vi "Purge Water Sequence SM.vi"(0 "Degree Setting":dbl=58.0, 1 "Equipment":T4={"COM Port"="COM9", "MW100"="MW100", "AG34970"="A-34972A", "Chamber"="WT500"}, 2 "Semiphore":T3, 5 "Flow rate setting":dbl=1.5, 7 "Temp Band(+/- F)":dbl=2.0, 9 "Valve Bank":u16(ring) items=["A", "B", "C", "D"], 11 "Error In":errorcluster, 12 "Flow Chart Ref":refnum<vi>, 13 "Temp Chart Ref":refnum<vi>, 14 "Test Condition":T1=enum."Global, Purge") -> (3 "Failed to Start Count":dbl, 4 "Downspout Flow":dbl=2.9, 6 "Downspout Temp":dbl=57.8, 8 "Flow rate setting out":dbl=2.250000000000002, 10 "Temp Setting Out":dbl=61.459999999999994, 15 "Error Out":errorcluster)   [LabVIEW 2012]
uses:
  EquipReferences.ctl
  Cluster Purge Settings.ctl
  TestedFlowratesScenarios.ctl
  ChannelSettings.ctl
  ValveBankPositions.ctl
  Intellifaucet/Intellfaucet Mode.ctl
  HEWH Error Enumeration.ctl
  Global HEWH.vi
panel:
  in  "Stop Chart":bool
  in  "Chart Data":bool
  out "Cold Flow":dbl[](array[numeric])
  in  "Purge Min Time":u32=30
  in  "Failed to Start Limit":dbl=5.0
  out "Output (Percent,GPM)":dbl
  in  "stop":bool
  in  "Ramp Down Array":dbl[](array[numeric])=[2.7, 2.5, 2.3, 2.1, 1.9, 1.7, 1.5, 1.3, 1.1, 0.9, 0.8]
  in  "Purge Settings Cluster":T2={"Temp SettleTimeLimit(S)"=120.0, "Steady State Persist Time(mS)"=30000, "Purge Min Time"=30, "Flow SettleTimeLimit(S)"=120.0, "Flow Adjust Time (3s)"=1.5, "Flow Band (+/-GPM)"=0.25, "Proportional Control Adjust Rate"=0.2}
  out "FlowSetTime":dbl=46.09375
  out "FlowSetStartTime":dbl=60.796875
  out "Settle Time Start":dbl format="%.2f"
  out "FlowErrors":bool[](array[boolean])=[TRUE, TRUE, TRUE, TRUE, TRUE, TRUE, TRUE, TRUE, TRUE, TRUE, TRUE, TRUE, TRUE, TRUE, TRUE, TRUE, TRUE, TRUE, TRUE, TRUE, TRUE, TRUE, TRUE, TRUE, TRUE, TRUE, TRUE, TRUE, TRUE, TRUE, TRUE, TRUE, TRUE, TRUE, TRUE, TRUE, TRUE, TRUE, TRUE, TRUE]
  out "TempErrors":bool[](array[boolean])=[TRUE, TRUE, TRUE, TRUE, TRUE, TRUE, TRUE, TRUE, TRUE, TRUE, TRUE, TRUE, TRUE, TRUE, TRUE, TRUE, TRUE, TRUE, TRUE, TRUE, TRUE, TRUE, TRUE, TRUE, TRUE, TRUE, TRUE, TRUE, TRUE, TRUE, TRUE, TRUE, TRUE, TRUE, TRUE, TRUE, TRUE, TRUE, TRUE, TRUE]
  out "TempSet Time (sec)":dbl=60.015625 format="%.2f"
  in  "Sample Period(mS)":u32=500
  in  "Steady State Persist Time(mS)":u32=20000
  in  "Flow Adjust Time (3s)":dbl=2.0
  in  "Flow SettleTimeLimit(S)":dbl=300.0
  out "Downspout Flow Chart":dbl(graph)=2.9
  out "Current State":string="Finish"
  out "Downspout Temp Chart":dbl(graph)=57.8
  out "-E":dbl=0.10000000000000009
  in  "Proportional Control Adjust Rate":dbl=0.1
  in  "Temp SettleTimeLimit(S)":dbl=300.0
  in  "Flow Band (+/-GPM)":dbl=0.25
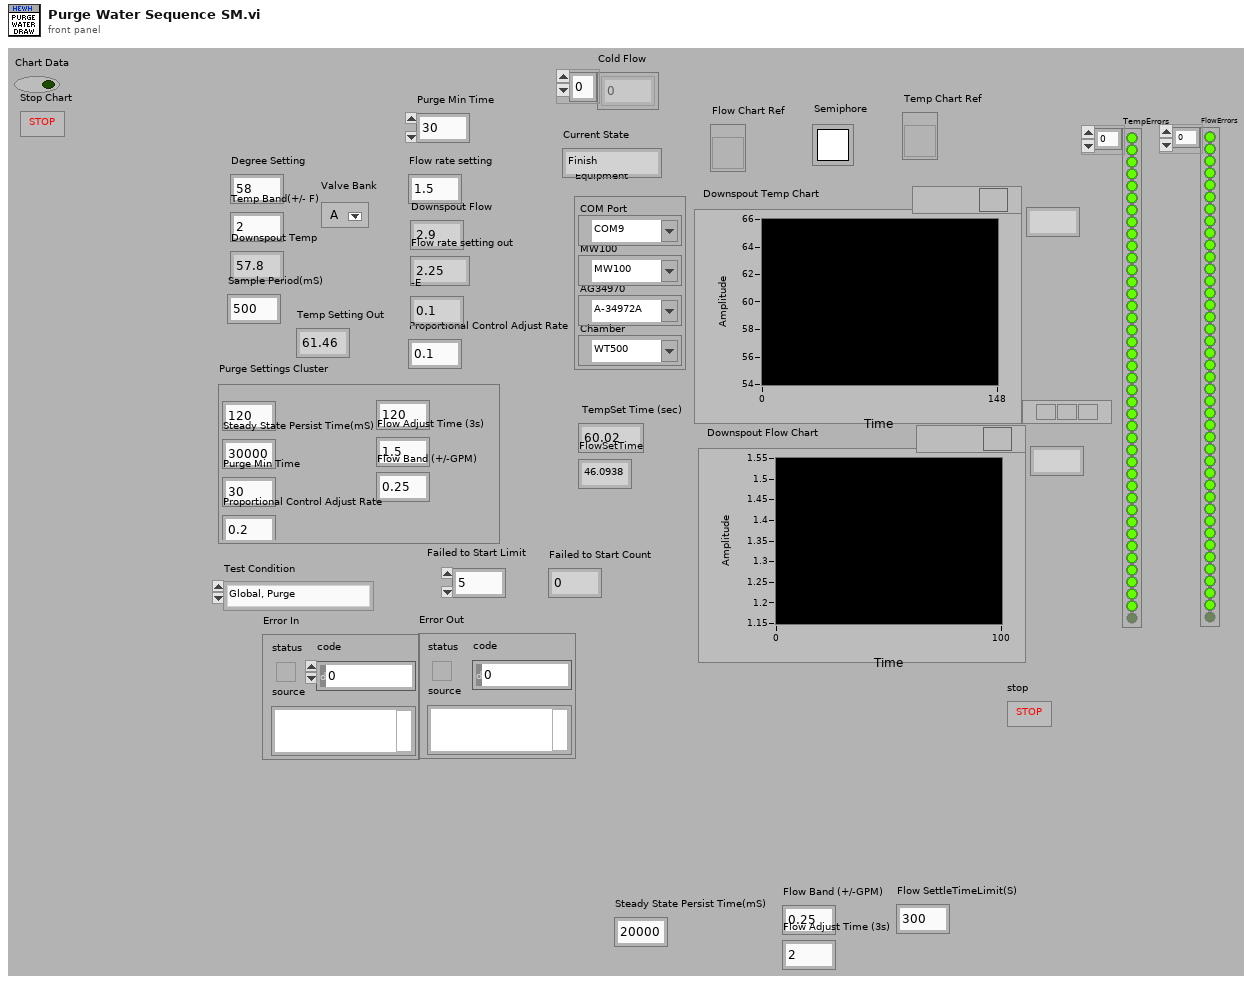
[diagram p1: front panel]
types:
  T1 = typedef "TestedFlowratesScenarios.ctl" = enum16{"DRK500,Station1", "DRK375,Lab", "SRK500,Station1,5GPM FR", "DRK375,STATION3,1/2\"HOSE", "DRK500,Station1,downspout", "DRK375,Station3,thruEcocute", "DRK375,Station3,purge", "Build2,2B,Purge", "Global, Purge", "Global, Tank"}
  T2 = typedef "Cluster Purge Settings.ctl" = cluster{"Temp SettleTimeLimit(S)":dbl, "Steady State Persist Time(mS)":u32, "Purge Min Time":i32, "Flow SettleTimeLimit(S)":dbl, "Flow Adjust Time (3s)":dbl, "Flow Band (+/-GPM)":dbl, "Proportional Control Adjust Rate":dbl}
  T3 = typedef "Semaphore RefNum" = refnum<k1>
  T4 = typedef "EquipReferences.ctl" = cluster{"COM Port":refnum<visa-resource-name>, "MW100":refnum<visa-resource-name>, "AG34970":refnum<visa-resource-name>, "Chamber":refnum<visa-resource-name>}
  T5 = typedef "ValveBankPositions.ctl" = enum16{"Heating", "Purge", "Resting", "Draw"}
  T6 = typedef "HEWH Error Enumeration.ctl" = enum16{"No Error", "GEA2 Send ACK Mismatch", "GEA2 STX", "GEA2 ETX", "GEA2 CRC Mismatch", "GEA2 ReadACK", "RTD In Range Error", "Fail Mean Tank Temp", "No Flow Config Data Found", "Failed Flow During Purge", "Temp During Purge", "Confirm IF Stop Fail", "Init Draw: TC_1 Out of Range", "Flow = 0 During Draw after 20s"}
  T7 = typedef "Intellfaucet Mode.ctl" = enum16{"Adjust Temp", "Adjust Flow", "Start Flow", "Stop Flow"}
  T8 = typedef "ChannelSettings.ctl" = u32
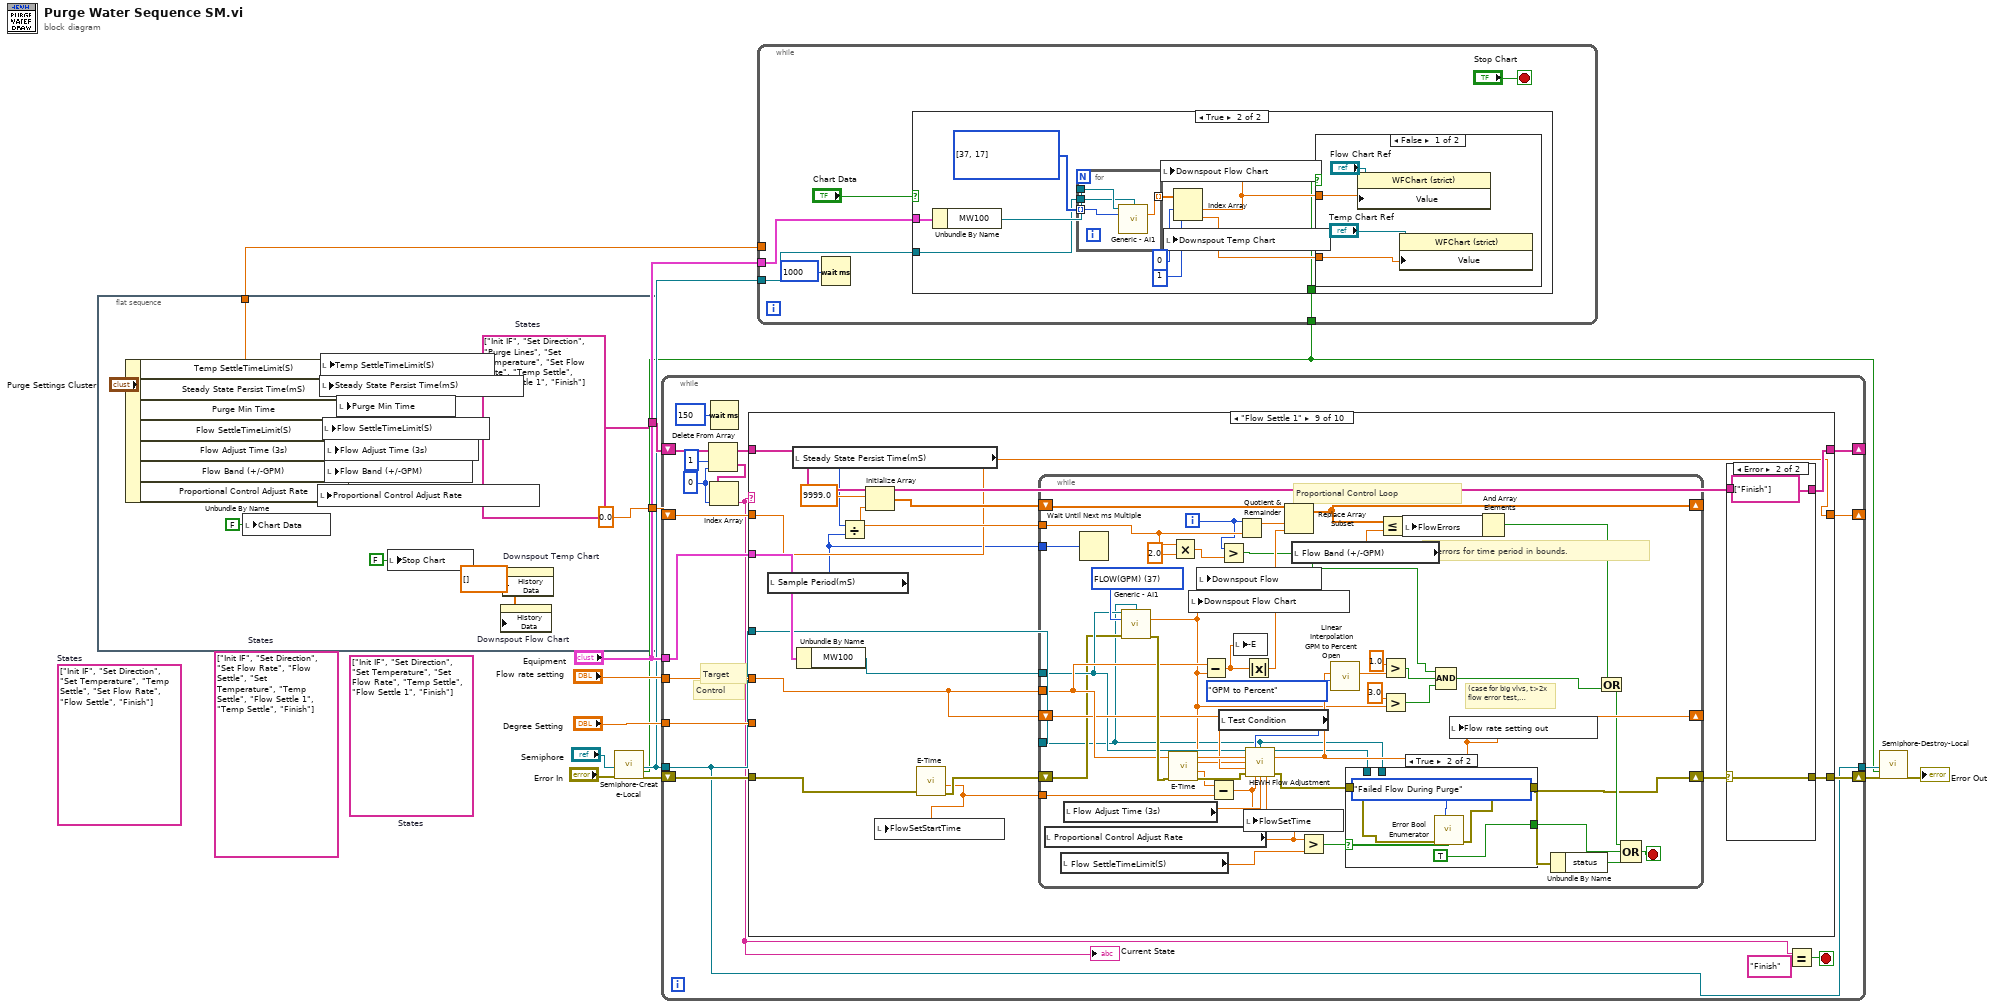
[diagram p0: block diagram]
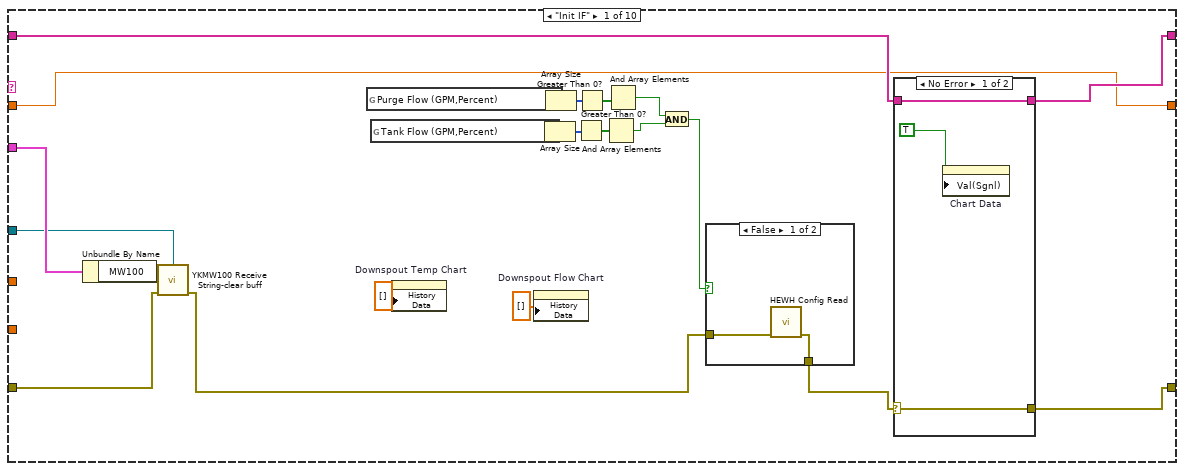
[diagram p4: hidden frame]
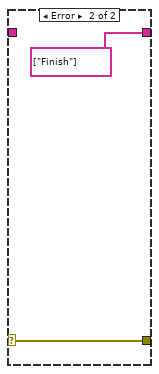
[diagram p6: hidden frame]
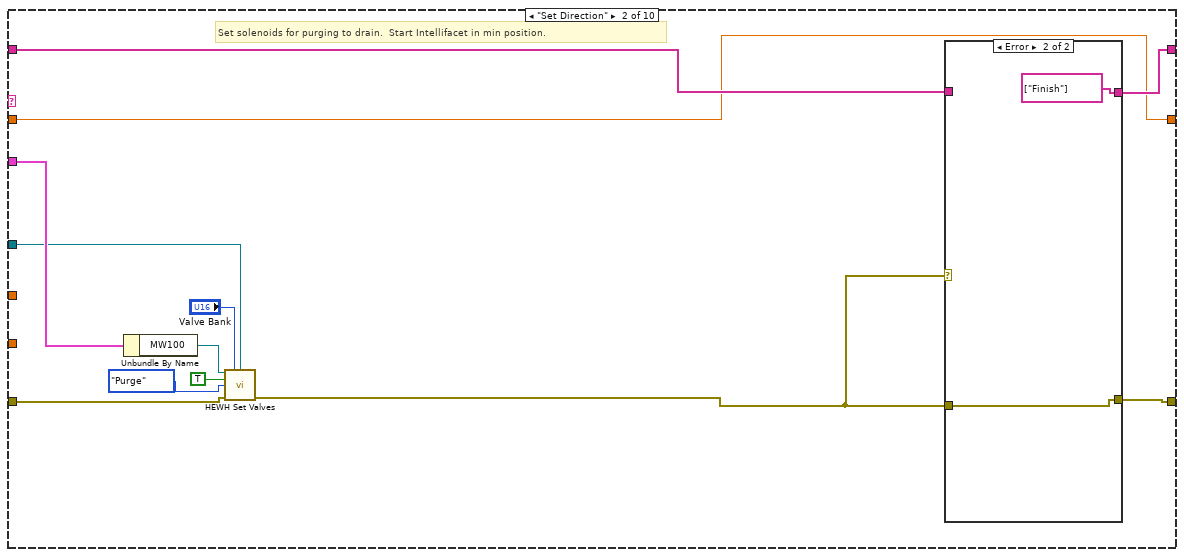
[diagram p7: hidden frame]
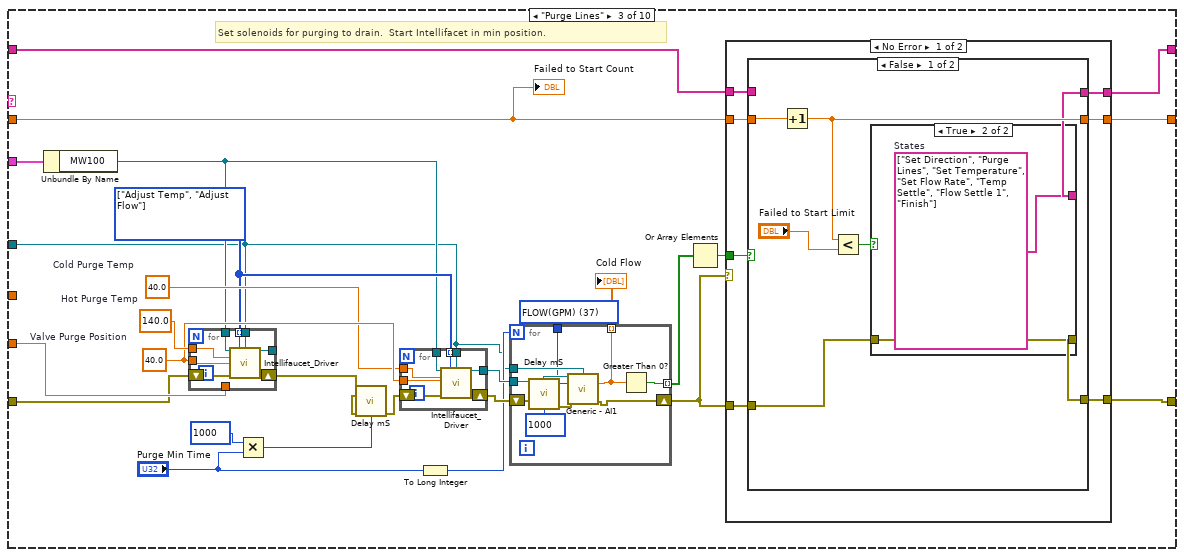
[diagram p9: hidden frame]
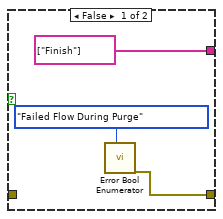
[diagram p10: hidden frame]
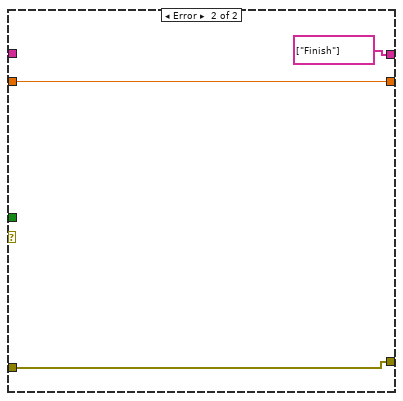
[diagram p12: hidden frame]
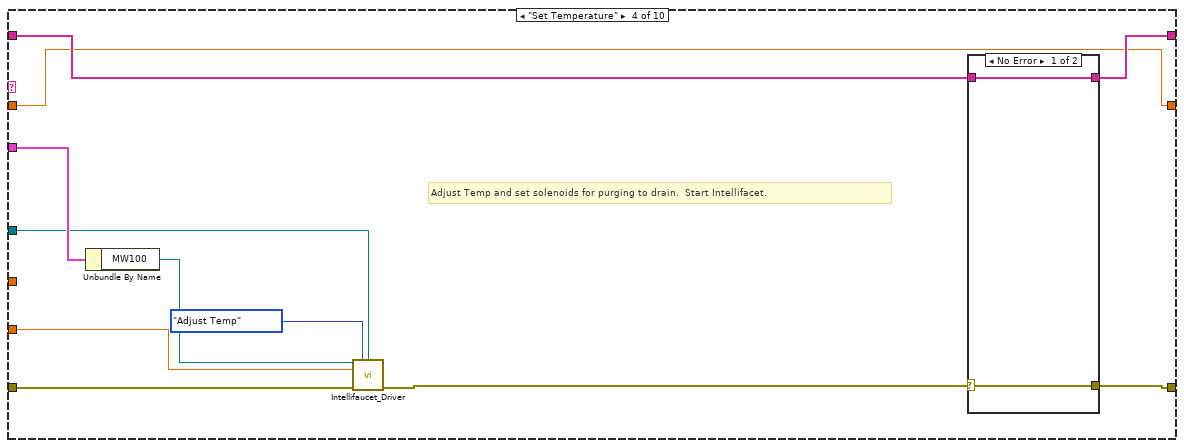
[diagram p13: hidden frame]
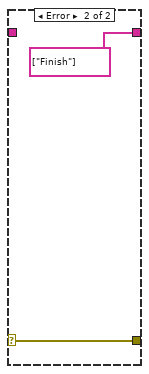
[diagram p14: hidden frame]
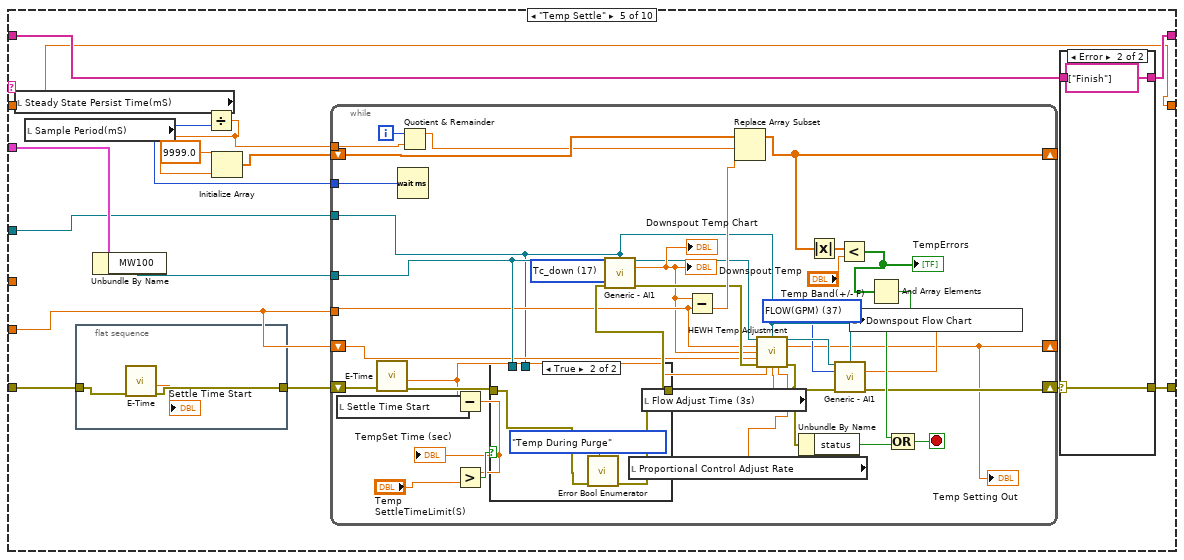
[diagram p15: hidden frame]
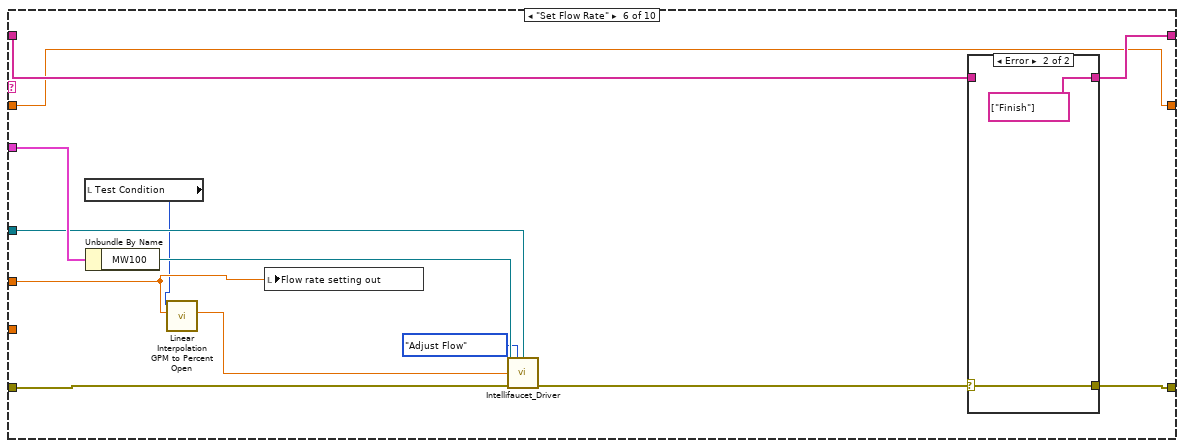
[diagram p18: hidden frame]
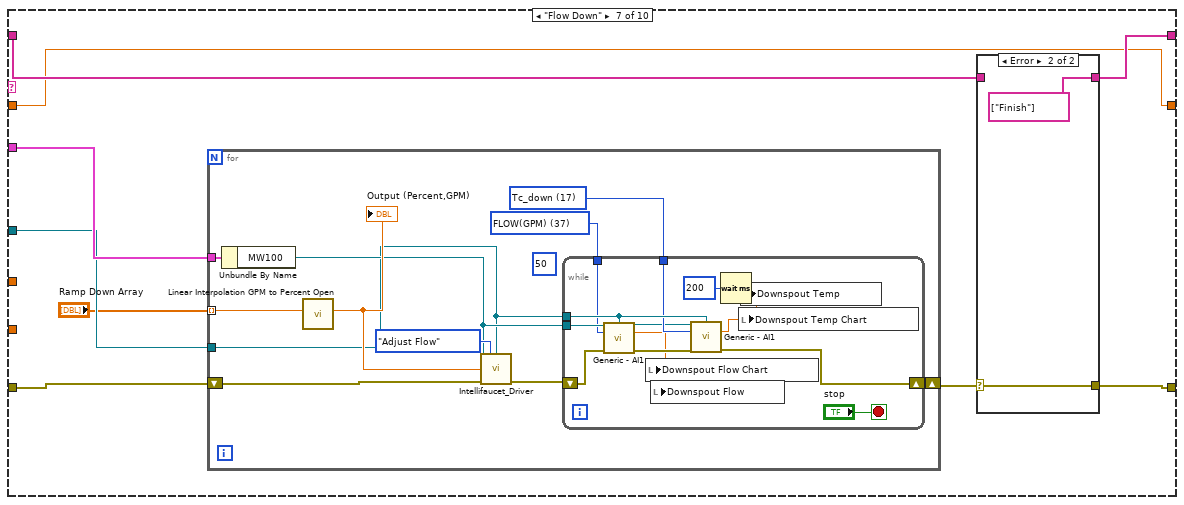
[diagram p20: hidden frame]
diagram:
  (unwired) string[] ["Init IF", "Set Direction", "Set Temperature", "Set Flow Rate", "Temp Settle", "Flow Settle 1", "Finish"]  # States
  (unwired) string[] ["Init IF", "Set Direction", "Set Flow Rate", "Flow Settle", "Set Temperature", "Temp Settle", "Flow Settle 1", "Temp Settle", "Finish"]  # States
  (unwired) string[] ["Init IF", "Set Direction", "Set Temperature", "Temp Settle", "Set Flow Rate", "Flow Settle", "Finish"]  # States
  n1 = flat-sequence {
    tunnel: [w19] -> w14
    tunnel: [0.0] -> w5
    tunnel: [w15] -> w1
    frame #0 {
      w19 = string[] ["Init IF", "Set Direction", "Purge Lines", "Set Temperature", "Set Flow Rate", "Temp Settle", "Flow Settle 1", "Finish"]  # States
      w20 = dbl[] [] ("History Data")
      n2 = Unbundle By Name("Purge Settings Cluster") -> ("Temp SettleTimeLimit(S)"=w15:dbl, "Steady State Persist Time(mS)"=w27:u32, "Purge Min Time"=w18:i32, "Flow SettleTimeLimit(S)"=w26:dbl, "Flow Adjust Time (3s)"=w25:dbl, "Flow Band (+/-GPM)"=w24:dbl, "Proportional Control Adjust Rate"=w23:dbl)
      n3 = local write "Chart Data"(FALSE ("Chart Data")) -> ()
      n4 = local write "Proportional Control Adjust Rate"(w23) -> ()
      n5 = local write "Steady State Persist Time(mS)"(w27) -> ()
      n6 = local write "Temp SettleTimeLimit(S)"(w15) -> ()
      n7 = local write "Flow SettleTimeLimit(S)"(w26) -> ()
      n8 = local write "Flow Adjust Time (3s)"(w25) -> ()
      n9 = local write "Flow Band (+/-GPM)"(w24) -> ()
      n10 = local write "Purge Min Time"(w18) -> ()
      n11 = local write "Stop Chart"(FALSE ("Stop Chart")) -> ()
      n12 = property on="Downspout Flow Chart" class="WFChart (strict)"("History Data"=w20) -> ()  [unwired: 2 in, 2 out]
      n13 = property on="Downspout Temp Chart" class="WFChart (strict)"("History Data"=w20) -> ()  [unwired: 2 in, 2 out]
    }
  }
  n14 = call "Semiphore-Create-Local.vi"("Semiphore"="Semiphore", "error in (no error)"="Error In") -> ("semaphore"=w3:T3, "Local?"=w2:bool, "error out"=w10:errorcluster)  [unwired: 15 in]
  n15 = while {
    shift-right: [w41] -> _
    shift-left: w14 -> [w45]
    shift-right: [w38] -> w9
    shift-left: w10 -> [w37]
    tunnel: "Equipment" -> [w30]
    tunnel: "Degree Setting" -> [w34]
    tunnel: "Flow rate setting" -> [w33]
    tunnel: w3 -> [w29]
    tunnel: [w29] -> w7
    shift-right: [w32] -> _
    shift-left: w5 -> [w31]
    stop <- w36 stop-if-true
    w42 = 0 ("index")
    # "Control"
    # "Target"
    n16 = Delete From Array(array=w45, length=1, index=w42) -> (deleted portion=w43:string[], array with subset deleted=w40:string[])
    n17 = Index Array(array=w43, index=w42) -> (element=w28:string)
    "Current State" <- w28
    n18 = Wait (ms)(milliseconds to wait=u32 150) -> ()  [unwired: 1 out]
    n19 = case shown="\"Flow Settle 1\"" w28 {
      tunnel: [w61 w85 w116 w176 w195 w257 w270 w315 w386 w451] -> w41
      tunnel: w40 -> [w62 w86 w117 w177 w196 w258 w271 w316 w387 w450]
      tunnel: [w59 w84 w115 w175 w193 w256 w269 w313 w384 w449] -> w38
      tunnel: w37 -> [w64 w83 w109 w174 w190 w254 w267 w311 w382 w448]
      tunnel: w30 -> [w66 w82 w92 w178 w198 w259 w272 w317 w388 _]
      tunnel: w34 -> [_ _ w110 w173 w184 _ _ _ _ _]
      tunnel: w33 -> [_ _ _ _ _ w248 _ w310 w372 _]
      tunnel: w29 -> [w63 w79 w91 w169 w192 w252 w266 w303 w377 _]
      tunnel: [w60 w76 w113 w168 w183 w249 w265 w301 w375 w447] -> w32
      tunnel: w31 -> [w60 w76 w111 w168 w183 w249 w265 w301 w375 w447]
      frame "Init IF" {
        n20 = Unbundle By Name(w66) -> ("MW100"=w65:refnum<visa-resource-name>)
        n21 = call "YKMW100 Receive String-clear buff.vi"("VISA session"=w65, "Semiphore"=w63, "error in (no error)"=w64) -> ("error out"=w48:errorcluster)  [unwired: 10 in, 2 out]
        n22 = global read "Global HEWH.vi" "Purge Flow (GPM,Percent)"() -> (w58:dbl[][])
        n23 = global read "Global HEWH.vi" "Tank Flow (GPM,Percent)"() -> (w57:dbl[][])
        n24 = property on="Downspout Temp Chart" class="WFChart (strict)"("History Data"=dbl[] []) -> ()  [unwired: 2 in, 2 out]
        n25 = property on="Downspout Flow Chart" class="WFChart (strict)"("History Data"=dbl[] []) -> ()  [unwired: 2 in, 2 out]
        n26 = Array Size(array=w57) -> (size(s)=w55:i32[])
        n27 = Array Size(array=w58) -> (size(s)=w56:i32[])
        n28 = Greater Than 0?(x=w55) -> (x > 0?=w53:bool[])
        n29 = Greater Than 0?(x=w56) -> (x > 0?=w54:bool[])
        n30 = And Array Elements(Boolean array=w53) -> (logical AND=w51:bool)
        n31 = And Array Elements(Boolean array=w54) -> (logical AND=w52:bool)
        n32 = And(x=w52, y=w51) -> (x .and. y?=w50:bool)
        n33 = case shown="False" w50 {
          tunnel: w48 -> [w68 w69]
          tunnel: [w67 w69] -> w49
          frame False {
            n34 = call "HEWH Config Read.vi"("error in (no error)"=w68) -> ("error out"=w67:errorcluster)  [unwired: 13 in, 1 out]
          }
          frame True {
          }
        }
        n35 = case shown="No Error" w49 {
          selector: w49 -> [w71 w74]
          tunnel: [w72 string[] ["Finish"] ("States")] -> w61
          tunnel: w62 -> [w72 _]
          tunnel: [w71 w74] -> w59
          frame No Error {
            n36 = property on="Chart Data" class="Bool (strict)"("Val(Sgnl)"=TRUE ("Chart Data")) -> ()  [unwired: 2 in, 2 out]
          }
          frame Error {
          }
        }
      }
      frame "Set Direction" {
        # "Set solenoids for purging to drain.  Start Intellifacet in min position."
        n37 = Unbundle By Name(w82) -> ("MW100"=w81:refnum<visa-resource-name>)
        n38 = call "HEWH Set Valves.vi"("VISA session"=w81, "Valve Bank"="Valve Bank", "Semiphore"=w79, "Expansion Tank?"=TRUE, "Valve Bank Setting"=ValveBankPositions."Purge", "Error In"=w83) -> ("Error Out"=w75:errorcluster)  [unwired: 8 in, 1 out]
        n39 = case shown="Error" w75 {
          tunnel: w86 -> [w88 _]
          tunnel: [w88 string[] ["Finish"] ("States")] -> w85
          tunnel: [w87 w89] -> w84
          tunnel: w75 -> [w87 w89]
          frame No Error {
          }
          frame Error {
          }
        }
      }
      frame "Purge Lines" {
        w99 = 40.0  # Cold Purge Temp
        w100 = 40.0  # Valve Purge Position
        w108 = 140.0  # Hot Purge Temp
        w98 = T7[] [enum."Adjust Temp", enum."Adjust Flow"] items=["Adjust Temp", "Adjust Flow", "Start Flow", "Stop Flow"]
        w114 = T8 37 items=["4-20_OUT", "Pres_HI1", "Pres_HI2", "Pres_LOW", "Pres_PIN", "HEATER_TOP", "HEATER_BOT", "T_Shell", "FLOWMETER", "WATT_SENSE", "WH_TICK", "Tc_1", "Tc_2", "Tc_3", "Tc_4", "Tc_5", "Tc_6", "Tc_down", "T_Shell_2", "T_Shell_3", "T_Shell_4", "RTD_IN", "RTD_OUT", "RTD_AMB", "INTF_TEMPFLO", "INTF_READY", "INTF_START", "INTF_STOP", "DRM_LOW", "DRM_HIGH", "PWR_MAIN", "VLV_DUMP", "VLV_OUT", "VLV_IN", "WATT_HOURS", "FLOW(SAMPLE)", "GALLONS", "FLOW(GPM)"] ("Channel_Enum")
        # "Set solenoids for purging to drain.  Start Intellifacet in min position."
        n40 = Unbundle By Name(w92) -> ("MW100"=w93:refnum<visa-resource-name>)
        n41 = for {
          tunnel: [w133] -> _
          tunnel: w98 -> [w132] mode=indexing
          tunnel: w91 -> [w129]
          shift-right: [w131] -> w107
          shift-left: w109 -> [w130]
          tunnel: w93 -> [w128]
          tunnel: w110 -> [_]
          tunnel: w100 -> [w126]
          tunnel: w108 -> [w127]
          n42 = call "Intellifaucet_Driver.vi"("VISA session"=w128, "Mode"=w132, "Semiphore"=w129, "Temperature(F)"=w127, "Percent Flow"=w126, "Error In"=w130) -> ("VISA session out"=w133:refnum<visa-resource-name>, "Error Out"=w131:errorcluster)  [unwired: 8 in]
        }
        n43 = Multiply(x=u32 1000 ("milliseconds to wait"), y="Purge Min Time") -> (x*y=w104:u32)
        n44 = call "Delay mS.vi"("Error In"=w107, "milliseconds to wait"=w104) -> ("Error Out"=w103:errorcluster)  [unwired: 13 in]
        n45 = for {
          tunnel: [w125] -> w101
          tunnel: w98 -> [w124] mode=indexing
          tunnel: w91 -> [w121]
          shift-right: [w123] -> w102
          shift-left: w103 -> [w122]
          tunnel: w93 -> [w120]
          tunnel: w100 -> [w119]
          tunnel: w99 -> [w118]
          n46 = call "Intellifaucet_Driver.vi"("VISA session"=w120, "Mode"=w124, "Semiphore"=w121, "Temperature(F)"=w118, "Percent Flow"=w119, "Error In"=w122) -> ("VISA session out"=w125:refnum<visa-resource-name>, "Error Out"=w123:errorcluster)  [unwired: 8 in]
        }
        n47 = To Long Integer(number="Purge Min Time") -> (32bit integer=w97:i32)
        n48 = for {
          N: w97 -> [_]
          tunnel: w91 -> [w140]
          tunnel: w101 -> [w139]
          tunnel: w114 -> [w138]
          tunnel: [w137] -> w96 mode=indexing
          shift-right: [w136] -> w112
          shift-left: w102 -> [w142]
          tunnel: [w134] -> w94 mode=indexing
          n49 = call "Delay mS.vi"("Error In"=w142, "milliseconds to wait"=u32 1000) -> ("Error Out"=w141:errorcluster)  [unwired: 13 in]
          n50 = call "Generic - AI1.vi"("MW100"=w139, "Semiphore"=w140, "Channel_Enum"=w138, "Error In"=w141) -> ("Value"=w134:dbl, "Error Out"=w136:errorcluster)  [unwired: 9 in, 1 out]
          n51 = Greater Than 0?(x=w134) -> (x > 0?=w137:bool)
        }
        "Cold Flow" <- w94
        n52 = Or Array Elements(Boolean array=w96) -> (logical OR=w95:bool)
        n53 = case shown="No Error" w112 {
          tunnel: w117 -> [w149 _]
          tunnel: [w148 string[] ["Finish"] ("States")] -> w116
          tunnel: [w147 w165] -> w115
          tunnel: w112 -> [w146 w165]
          tunnel: w95 -> [w145 _]
          tunnel: [w144 w166] -> w113
          tunnel: w111 -> [w143 w166]
          frame No Error {
            n54 = case shown="False" w145 {
              tunnel: w149 -> [_ w164]
              tunnel: [w152 w164] -> w148
              tunnel: [w151 w162] -> w147
              tunnel: w146 -> [w150 w162]
              tunnel: [w155 w163] -> w144
              tunnel: w143 -> [w156 w163]
              frame False {
                n55 = Increment(x=w156) -> (x+1=w155:dbl)
                n56 = Less?(x=w155, y="Failed to Start Limit") -> (x < y?=w153:bool)
                n57 = case shown="True" w153 {
                  tunnel: [string[] ["Finish"] ("States") w160] -> w152
                  tunnel: [w158 w161] -> w151
                  tunnel: w150 -> [_ w161]
                  frame False {
                    n58 = call "Error Bool Enumerator.vi"("Error Enum"=HEWH_Error_Enumeration."Failed Flow During Purge") -> ("Error Out"=w158:errorcluster)  [unwired: 8 in]
                  }
                  frame True {
                    w160 = string[] ["Set Direction", "Purge Lines", "Set Temperature", "Set Flow Rate", "Temp Settle", "Flow Settle 1", "Finish"]  # States
                  }
                }
              }
              frame True {
              }
            }
          }
          frame Error {
          }
        }
        "Failed to Start Count" <- w111
      }
      frame "Set Temperature" {
        # "Adjust Temp and set solenoids for purging to drain.  Start Intellifacet."
        n59 = Unbundle By Name(w178) -> ("MW100"=w171:refnum<visa-resource-name>)
        n60 = call "Intellifaucet_Driver.vi"("VISA session"=w171, "Mode"=Intellfaucet_Mode."Adjust Temp", "Semiphore"=w169, "Temperature(F)"=w173, "Error In"=w174) -> ("Error Out"=w170:errorcluster)  [unwired: 9 in, 1 out]
        n61 = case shown="No Error" w170 {
          selector: w170 -> [w179 w182]
          tunnel: [w180 string[] ["Finish"] ("States")] -> w176
          tunnel: w177 -> [w180 _]
          tunnel: [w179 w182] -> w175
          frame No Error {
          }
          frame Error {
          }
        }
      }
      frame "Temp Settle" {
        n62 = local read "Steady State Persist Time(mS)"() -> (w189:u32)
        n63 = local read "Sample Period(mS)"() -> (w185:u32)
        n64 = flat-sequence {
          tunnel: [w201] -> w191
          tunnel: w190 -> [w200]
          frame #0 {
            n65 = call "E-Time.vi"("error in (no error)"=w200) -> ("error out"=w201:errorcluster, "Elapsed Time (sec)"=→"Settle Time Start":dbl)  [unwired: 8 in, 1 out]
          }
        }
        n66 = Unbundle By Name(w198) -> ("MW100"=w197:refnum<visa-resource-name>)
        n67 = Divide(x=w189, y=w185) -> (x/y=w187:dbl)
        n68 = Initialize Array(9999.0 ("element"), w187) -> (w186:dbl[])
        n69 = while {
          tunnel: w197 -> [w221]
          tunnel: w184 -> [w219]
          shift-right: [w212] -> w194
          shift-left: w191 -> [w227]
          tunnel: w192 -> [w210]
          tunnel: w187 -> [w237]
          shift-right: [w233] -> _
          shift-left: w186 -> [w236]
          tunnel: w185 -> [w228]
          shift-right: [w206] -> _
          shift-left: w184 -> [w217]
          i -> [w238]
          stop <- w242 stop-if-true
          w208 = T8 37 items=["4-20_OUT", "Pres_HI1", "Pres_HI2", "Pres_LOW", "Pres_PIN", "HEATER_TOP", "HEATER_BOT", "T_Shell", "FLOWMETER", "WATT_SENSE", "WH_TICK", "Tc_1", "Tc_2", "Tc_3", "Tc_4", "Tc_5", "Tc_6", "Tc_down", "T_Shell_2", "T_Shell_3", "T_Shell_4", "RTD_IN", "RTD_OUT", "RTD_AMB", "INTF_TEMPFLO", "INTF_READY", "INTF_START", "INTF_STOP", "DRM_LOW", "DRM_HIGH", "PWR_MAIN", "VLV_DUMP", "VLV_OUT", "VLV_IN", "WATT_HOURS", "FLOW(SAMPLE)", "GALLONS", "FLOW(GPM)"] ("Channel_Enum")
          w240 = T8 17 items=["4-20_OUT", "Pres_HI1", "Pres_HI2", "Pres_LOW", "Pres_PIN", "HEATER_TOP", "HEATER_BOT", "T_Shell", "FLOWMETER", "WATT_SENSE", "WH_TICK", "Tc_1", "Tc_2", "Tc_3", "Tc_4", "Tc_5", "Tc_6", "Tc_down", "T_Shell_2", "T_Shell_3", "T_Shell_4", "RTD_IN", "RTD_OUT", "RTD_AMB", "INTF_TEMPFLO", "INTF_READY", "INTF_START", "INTF_STOP", "DRM_LOW", "DRM_HIGH", "PWR_MAIN", "VLV_DUMP", "VLV_OUT", "VLV_IN", "WATT_HOURS", "FLOW(SAMPLE)", "GALLONS", "FLOW(GPM)"] ("Channel_Enum")
          n70 = local read "Settle Time Start"() -> (w223:dbl)
          n71 = call "E-Time.vi"("error in (no error)"=w227) -> ("error out"=w226:errorcluster, "Elapsed Time (sec)"=w216:dbl)  [unwired: 8 in, 1 out]
          n72 = Wait (ms)(milliseconds to wait=w228) -> ()  [unwired: 1 out]
          n73 = Quotient & Remainder(x=w238, y=w237) -> (x-y*floor(x/y)=w235:dbl)  [unwired: 1 out]
          n74 = Subtract(x=w216, y=w223) -> (x-y=w222:dbl)
          "TempSet Time (sec)" <- w222
          n75 = Greater?(x=w222, y="Temp SettleTimeLimit(S)") -> (0:w241:bool)
          n76 = case shown="True" w241 {
            tunnel: w226 -> [w243 w244]
            tunnel: [w243 w245] -> w225
            tunnel: w210 -> [_ _]
            tunnel: w221 -> [_ _]
            frame False {
            }
            frame True {
              n77 = call "Error Bool Enumerator.vi"("Error Enum"=HEWH_Error_Enumeration."Temp During Purge", "Error In"=w244) -> ("Error Out"=w245:errorcluster)  [unwired: 7 in]
            }
          }
          n78 = call "Generic - AI1.vi"("MW100"=w221, "Semiphore"=w210, "Channel_Enum"=w240, "Error In"=w225) -> ("dup VISA session"=w215:refnum<visa-resource-name>, "Value"=w218:dbl, "Error Out"=w220:errorcluster)  [unwired: 9 in]
          "Downspout Temp" <- w218
          "Downspout Temp Chart" <- w218
          n79 = local read "Proportional Control Adjust Rate"() -> (w213:dbl)
          n80 = local read "Flow Adjust Time (3s)"() -> (w214:dbl)
          n81 = Subtract(x=w218, y=w219) -> (x-y=w234:dbl)
          n82 = Replace Array Subset(array=w236, new element=w234, index=w235) -> (w233:dbl[])
          n83 = call "HEWH Temp Adjustment.vi"("VISA session"=w215, "Semiphore"=w210, "Degrees Target(58)"=w219, "Degrees reading"=w218, "Degrees setting In"=w217, "Error In"=w220, "Elapsed Time (sec)"=w216, "Temp Adjust Time (3s)"=w214, "K(0.1)"=w213) -> ("VISA session out"=w209:refnum<visa-resource-name>, "Degree setting Out"=w206:dbl, "Error Out"=w211:errorcluster)  [unwired: 4 in]
          "Temp Setting Out" <- w206
          n84 = Unbundle By Name(w211) -> ("status"=w224:bool)
          n85 = Absolute Value(x=w233) -> (abs(x)=w232:dbl[])
          n86 = call "Generic - AI1.vi"("MW100"=w209, "Semiphore"=w210, "Channel_Enum"=w208, "Error In"=w211) -> ("Value"=w207:dbl, "Error Out"=w212:errorcluster)  [unwired: 9 in, 1 out]
          n87 = Less?(x=w232, y="Temp Band(+/- F)") -> (x < y?=w230:bool[])
          "TempErrors" <- w230
          n88 = local write "Downspout Flow Chart"(w207) -> ()
          n89 = And Array Elements(Boolean array=w230) -> (logical AND=w229:bool)
          n90 = Compound Arithmetic op=OR(w229, w224) -> (w242:bool)
        }
        n91 = case shown="Error" w194 {
          selector: w194 -> [w202 w205]
          tunnel: [w203 string[] ["Finish"] ("States")] -> w195
          tunnel: w196 -> [w203 _]
          tunnel: [w202 w205] -> w193
          frame No Error {
          }
          frame Error {
          }
        }
      }
      frame "Set Flow Rate" {
        n92 = local read "Test Condition"() -> (w247:T1)
        n93 = Unbundle By Name(w259) -> ("MW100"=w253:refnum<visa-resource-name>)
        n94 = call "Linear Interpolation GPM to Percent Open.vi"("Input (GPM,Percent)"=w248, "Configuration"=w247) -> ("Output (Percent,GPM)"=w250:dbl)  [unwired: 9 in]
        n95 = local write "Flow rate setting out"(w248) -> ()
        n96 = call "Intellifaucet_Driver.vi"("VISA session"=w253, "Mode"=Intellfaucet_Mode."Adjust Flow", "Semiphore"=w252, "Percent Flow"=w250, "Error In"=w254) -> ("Error Out"=w255:errorcluster)  [unwired: 9 in, 1 out]
        n97 = case shown="Error" w255 {
          selector: w255 -> [w260 w263]
          tunnel: [w261 string[] ["Finish"] ("States")] -> w257
          tunnel: w258 -> [w261 _]
          tunnel: [w260 w263] -> w256
          frame No Error {
          }
          frame Error {
          }
        }
      }
      frame "Flow Down" {
        n98 = for {
          tunnel: w272 -> [w283]
          tunnel: w266 -> [w277]
          shift-right: [w273] -> w268
          shift-left: w267 -> [w282]
          tunnel: "Ramp Down Array" -> [w279] mode=indexing
          w275 = T8 17 items=["4-20_OUT", "Pres_HI1", "Pres_HI2", "Pres_LOW", "Pres_PIN", "HEATER_TOP", "HEATER_BOT", "T_Shell", "FLOWMETER", "WATT_SENSE", "WH_TICK", "Tc_1", "Tc_2", "Tc_3", "Tc_4", "Tc_5", "Tc_6", "Tc_down", "T_Shell_2", "T_Shell_3", "T_Shell_4", "RTD_IN", "RTD_OUT", "RTD_AMB", "INTF_TEMPFLO", "INTF_READY", "INTF_START", "INTF_STOP", "DRM_LOW", "DRM_HIGH", "PWR_MAIN", "VLV_DUMP", "VLV_OUT", "VLV_IN", "WATT_HOURS", "FLOW(SAMPLE)", "GALLONS", "FLOW(GPM)"] ("Channel_Enum")
          w276 = T8 37 items=["4-20_OUT", "Pres_HI1", "Pres_HI2", "Pres_LOW", "Pres_PIN", "HEATER_TOP", "HEATER_BOT", "T_Shell", "FLOWMETER", "WATT_SENSE", "WH_TICK", "Tc_1", "Tc_2", "Tc_3", "Tc_4", "Tc_5", "Tc_6", "Tc_down", "T_Shell_2", "T_Shell_3", "T_Shell_4", "RTD_IN", "RTD_OUT", "RTD_AMB", "INTF_TEMPFLO", "INTF_READY", "INTF_START", "INTF_STOP", "DRM_LOW", "DRM_HIGH", "PWR_MAIN", "VLV_DUMP", "VLV_OUT", "VLV_IN", "WATT_HOURS", "FLOW(SAMPLE)", "GALLONS", "FLOW(GPM)"] ("Channel_Enum")
          (unwired) 50
          n99 = Unbundle By Name(w283) -> ("MW100"=w278:refnum<visa-resource-name>)
          n100 = call "Linear Interpolation GPM to Percent Open.vi"("Input (GPM,Percent)"=w279) -> ("Output (Percent,GPM)"=w280:dbl)  [unwired: 10 in]
          "Output (Percent,GPM)" <- w280
          n101 = call "Intellifaucet_Driver.vi"("VISA session"=w278, "Mode"=Intellfaucet_Mode."Adjust Flow", "Semiphore"=w277, "Percent Flow"=w280, "Error In"=w282) -> ("Error Out"=w274:errorcluster)  [unwired: 9 in, 1 out]
          n102 = while {
            tunnel: w278 -> [w295]
            tunnel: w277 -> [w294]
            tunnel: w276 -> [w292]
            tunnel: w275 -> [w291]
            shift-right: [w287] -> w273
            shift-left: w274 -> [w289]
            stop <- "stop" stop-if-true
            n103 = call "Generic - AI1.vi"("MW100"=w295, "Semiphore"=w294, "Channel_Enum"=w292, "Error In"=w289) -> ("dup VISA session"=w290:refnum<visa-resource-name>, "Value"=w286:dbl, "Error Out"=w288:errorcluster)  [unwired: 9 in]
            n104 = local write "Downspout Flow Chart"(w286) -> ()
            n105 = local write "Downspout Flow"(w286) -> ()
            n106 = call "Generic - AI1.vi"("MW100"=w290, "Semiphore"=w294, "Channel_Enum"=w291, "Error In"=w288) -> ("Value"=w285:dbl, "Error Out"=w287:errorcluster)  [unwired: 9 in, 1 out]
            n107 = Wait (ms)(milliseconds to wait=u32 200) -> ()  [unwired: 1 out]
            n108 = local write "Downspout Temp Chart"(w285) -> ()
            n109 = local write "Downspout Temp"(w285) -> ()
          }
        }
        n110 = case shown="Error" w268 {
          selector: w268 -> [w296 w299]
          tunnel: [w297 string[] ["Finish"] ("States")] -> w270
          tunnel: w271 -> [w297 _]
          tunnel: [w296 w299] -> w269
          frame No Error {
          }
          frame Error {
          }
        }
      }
      frame "Flow Settle" {
        # "Init flow rate"
        n111 = flat-sequence {
          tunnel: [w320] -> w312
          tunnel: w311 -> [w318]
          tunnel: w304 -> [_]
          tunnel: w303 -> [_]
          tunnel: [w319] -> w302
          frame #0 {
            n112 = property on="Downspout Flow Chart" class="WFChart (strict)"("History Data"=dbl[] []) -> ()  [unwired: 2 in, 2 out]
            n113 = call "E-Time.vi"("error in (no error)"=w318) -> ("error out"=w320:errorcluster, "Elapsed Time (sec)"=w319:dbl)  [unwired: 8 in, 1 out]
            "FlowSetStartTime" <- w319
          }
        }
        n114 = Unbundle By Name(w317) -> ("MW100"=w304:refnum<visa-resource-name>)
        n115 = Divide(x="Steady State Persist Time(mS)", y="Sample Period(mS)") -> (x/y=w307:dbl)
        n116 = Initialize Array(9999.0 ("element"), w307) -> (w306:dbl[])
        n117 = while {
          tunnel: w304 -> [w336]
          shift-right: [w354] -> w314
          shift-left: w312 -> [w331]
          tunnel: w310 -> [w352]
          shift-right: [w348] -> _
          shift-left: 0.0 ("Flow rate setting") -> [w351]
          tunnel: w303 -> [w330]
          tunnel: w307 -> [w345]
          tunnel: "Sample Period(mS)" -> [w342]
          shift-right: [w338] -> _
          shift-left: w306 -> [w343]
          tunnel: w302 -> [w333]
          i -> [w346]
          stop <- w361 stop-if-true
          w337 = T8 37 items=["4-20_OUT", "Pres_HI1", "Pres_HI2", "Pres_LOW", "Pres_PIN", "HEATER_TOP", "HEATER_BOT", "T_Shell", "FLOWMETER", "WATT_SENSE", "WH_TICK", "Tc_1", "Tc_2", "Tc_3", "Tc_4", "Tc_5", "Tc_6", "Tc_down", "T_Shell_2", "T_Shell_3", "T_Shell_4", "RTD_IN", "RTD_OUT", "RTD_AMB", "INTF_TEMPFLO", "INTF_READY", "INTF_START", "INTF_STOP", "DRM_LOW", "DRM_HIGH", "PWR_MAIN", "VLV_DUMP", "VLV_OUT", "VLV_IN", "WATT_HOURS", "FLOW(SAMPLE)", "GALLONS", "FLOW(GPM)"] ("Channel_Enum")
          # "Proportional Control Loop"
          n118 = Wait Until Next ms Multiple(millisecond multiple=w342) -> ()  [unwired: 1 out]
          n119 = call "Generic - AI1.vi"("MW100"=w336, "Semiphore"=w330, "Channel_Enum"=w337, "Error In"=w331) -> ("Value"=w335:dbl, "Error Out"=w353:errorcluster)  [unwired: 9 in, 1 out]
          "Downspout Flow" <- w335
          "Downspout Flow Chart" <- w335
          n120 = call "E-Time.vi"("error in (no error)"=w353) -> ("error out"=w350:errorcluster, "Elapsed Time (sec)"=w334:dbl)  [unwired: 8 in, 1 out]
          n121 = Subtract(x=w352, y=w335) -> (x-y=w357:dbl)
          "-E" <- w357
          n122 = Subtract(x=w334, y=w333) -> (x-y=w332:dbl)
          "FlowSetTime" <- w332
          n123 = Quotient & Remainder(x=w346, y=w345) -> (x-y*floor(x/y)=w344:dbl)  [unwired: 1 out]
          n124 = Absolute Value(x=w357) -> (abs(x)=w341:dbl)
          n125 = call "HEWH Flow Adjustment.vi"("VISA session"=w336, "Configuration"="Test Condition", "Semiphore"=w330, "GPM Target(3)"=w352, "GPM reading"=w335, "Flow rate setting In"=w351, "Error In"=w350, "Elapsed Time (sec)"=w332, "Flow Adjust Time (3s)"="Flow Adjust Time (3s)", "K(0.1)"="Proportional Control Adjust Rate") -> ("VISA session out"=w327:refnum<visa-resource-name>, "Flow rate setting Out"=w348:dbl, "Error Out"=w326:errorcluster)  [unwired: 3 in]
          "Flow rate setting out" <- w348
          n126 = Greater?(x=w332, y="Flow SettleTimeLimit(S)") -> (0:w359:bool)
          n127 = case shown="True" w359 {
            selector: w359 -> [w363 _]
            tunnel: w326 -> [w362 w370]
            tunnel: [w362 w366] -> w354
            tunnel: [w363 TRUE] -> w360
            tunnel: w327 -> [_ w369]
            tunnel: w330 -> [_ w368]
            tunnel: Intellfaucet_Mode."Stop Flow" ("Mode") -> [_ w367]
            frame False {
            }
            frame True {
              n128 = call "Intellifaucet_Driver.vi"("VISA session"=w369, "Mode"=w367, "Semiphore"=w368, "Error In"=w370) -> ("Error Out"=w365:errorcluster)  [unwired: 10 in, 1 out]
              n129 = call "Error Bool Enumerator.vi"("Error Enum"=HEWH_Error_Enumeration."Failed Flow During Purge", "Error In"=w365) -> ("Error Out"=w366:errorcluster)  [unwired: 7 in]
            }
          }
          n130 = Replace Array Subset(array=w343, new element=w341, index=w344) -> (w338:dbl[])
          n131 = Less Or Equal?(x=w338, y="Flow Band (+/-GPM)") -> (x <= y?=w340:bool[])
          "FlowErrors" <- w340
          n132 = Unbundle By Name(w354) -> ("status"=w355:bool)
          n133 = And Array Elements(Boolean array=w340) -> (logical AND=w339:bool)
          n134 = Compound Arithmetic op=OR(w339, w360, w355) -> (w361:bool)
        }
        n135 = case shown="Error" w314 {
          selector: w314 -> [w322 w325]
          tunnel: [w323 string[] ["Finish"] ("States")] -> w315
          tunnel: w316 -> [w323 _]
          tunnel: [w322 w325] -> w313
          frame No Error {
          }
          frame Error {
          }
        }
      }
      frame "Flow Settle 1" {
        n136 = local read "Sample Period(mS)"() -> (w373:u32)
        n137 = local read "Steady State Persist Time(mS)"() -> (w374:u32)
        n138 = Unbundle By Name(w388) -> ("MW100"=w378:refnum<visa-resource-name>)
        n139 = Divide(x=w374, y=w373) -> (x/y=w380:dbl)
        n140 = Initialize Array(9999.0 ("element"), w380) -> (w379:dbl[])
        n141 = call "E-Time.vi"("error in (no error)"=w382) -> ("error out"=w383:errorcluster, "Elapsed Time (sec)"=w376:dbl)  [unwired: 8 in, 1 out]
        n142 = local write "FlowSetStartTime"(w376) -> ()
        n143 = while {
          tunnel: w378 -> [w423]
          shift-right: [w393] -> w385
          shift-left: w383 -> [w420]
          tunnel: w372 -> [w433]
          shift-right: [w405] -> _
          shift-left: w372 -> [w432]
          tunnel: w377 -> [w394]
          tunnel: w380 -> [w400]
          tunnel: w373 -> [w428]
          shift-right: [w425] -> _
          shift-left: w379 -> [w429]
          tunnel: w376 -> [w421]
          i -> [w398]
          stop <- w438 stop-if-true
          w424 = T8 37 items=["4-20_OUT", "Pres_HI1", "Pres_HI2", "Pres_LOW", "Pres_PIN", "HEATER_TOP", "HEATER_BOT", "T_Shell", "FLOWMETER", "WATT_SENSE", "WH_TICK", "Tc_1", "Tc_2", "Tc_3", "Tc_4", "Tc_5", "Tc_6", "Tc_down", "T_Shell_2", "T_Shell_3", "T_Shell_4", "RTD_IN", "RTD_OUT", "RTD_AMB", "INTF_TEMPFLO", "INTF_READY", "INTF_START", "INTF_STOP", "DRM_LOW", "DRM_HIGH", "PWR_MAIN", "VLV_DUMP", "VLV_OUT", "VLV_IN", "WATT_HOURS", "FLOW(SAMPLE)", "GALLONS", "FLOW(GPM)"] ("Channel_Enum")
          # "(case for big vlvs, t>2x flow error test, \nvalve at 0, flow < 3gpm)"
          # "All errors for time period in bounds."
          # "Proportional Control Loop"
          n144 = local read "Proportional Control Adjust Rate"() -> (w416:dbl)
          n145 = local read "Flow SettleTimeLimit(S)"() -> (w415:dbl)
          n146 = local read "Flow Adjust Time (3s)"() -> (w417:dbl)
          n147 = Wait Until Next ms Multiple(millisecond multiple=w428) -> ()  [unwired: 1 out]
          n148 = call "Generic - AI1.vi"("MW100"=w423, "Semiphore"=w394, "Channel_Enum"=w424, "Error In"=w420) -> ("Value"=w402:dbl, "Error Out"=w434:errorcluster)  [unwired: 9 in, 1 out]
          n149 = call "E-Time.vi"("error in (no error)"=w434) -> ("error out"=w431:errorcluster, "Elapsed Time (sec)"=w422:dbl)  [unwired: 8 in, 1 out]
          n150 = Multiply(x=w400, y=2.0) -> (x*y=w397:dbl)
          n151 = local write "Downspout Flow Chart"(w402) -> ()
          n152 = local write "Downspout Flow"(w402) -> ()
          n153 = Subtract(x=w433, y=w402) -> (x-y=w418:dbl)
          n154 = Subtract(x=w422, y=w421) -> (x-y=w414:dbl)
          n155 = local read "Test Condition"() -> (w412:T1)
          n156 = Greater?(x=w398, y=w397) -> (0:w396:bool)
          n157 = local write "-E"(w418) -> ()
          n158 = Quotient & Remainder(x=w398, y=w400) -> (x-y*floor(x/y)=w430:dbl)  [unwired: 1 out]
          n159 = local write "FlowSetTime"(w414) -> ()
          n160 = Absolute Value(x=w418) -> (abs(x)=w427:dbl)
          n161 = call "HEWH Flow Adjustment.vi"("VISA session"=w423, "Configuration"=w412, "Semiphore"=w394, "GPM Target(3)"=w433, "GPM reading"=w402, "Flow rate setting In"=w432, "Error In"=w431, "Elapsed Time (sec)"=w414, "Flow Adjust Time (3s)"=w417, "K(0.1)"=w416) -> ("VISA session out"=w395:refnum<visa-resource-name>, "Flow rate setting Out"=w405:dbl, "Error Out"=w419:errorcluster)  [unwired: 3 in]
          n162 = Replace Array Subset(array=w429, new element=w427, index=w430) -> (w425:dbl[])
          n163 = local read "Flow Band (+/-GPM)"() -> (w413:dbl)
          n164 = Greater?(x=w414, y=w415) -> (0:w436:bool)
          n165 = call "Linear Interpolation GPM to Percent Open.vi"("Interp Direction"=enum16{"GPM to Percent", "Percent to GPM"}."GPM to Percent", "Input (GPM,Percent)"=w405) -> ("Output (Percent,GPM)"=w410:dbl)  [unwired: 9 in]
          n166 = case shown="True" w436 {
            selector: w436 -> [w440 _]
            tunnel: w419 -> [w439 w441]
            tunnel: [w439 w443] -> w393
            tunnel: [w440 TRUE] -> w437
            tunnel: w395 -> [_ _]
            tunnel: w394 -> [_ _]
            frame False {
            }
            frame True {
              n167 = call "Error Bool Enumerator.vi"("Error Enum"=HEWH_Error_Enumeration."Failed Flow During Purge", "Error In"=w441) -> ("Error Out"=w443:errorcluster)  [unwired: 7 in]
            }
          }
          n168 = Less Or Equal?(x=w425, y=w413) -> (x <= y?=w411:bool[])
          n169 = Greater?(x=1.0, y=w410) -> (0:w408:bool)
          n170 = Greater?(x=3.0, y=w402) -> (0:w406:bool)
          n171 = local write "FlowErrors"(w411) -> ()
          n172 = Compound Arithmetic op=AND(w396, w408, w406) -> (w401:bool)
          n173 = local write "Flow rate setting out"(w405) -> ()
          n174 = And Array Elements(Boolean array=w411) -> (logical AND=w426:bool)
          n175 = Unbundle By Name(w393) -> ("status"=w435:bool)
          n176 = Or(x=w426, y=w401) -> (x .or. y?=w404:bool)
          n177 = Compound Arithmetic op=OR(w404, w437, w435) -> (w438:bool)
        }
        n178 = case shown="Error" w385 {
          selector: w385 -> [w389 w392]
          tunnel: [w390 string[] ["Finish"] ("States")] -> w386
          tunnel: w387 -> [w390 _]
          tunnel: [w389 w392] -> w384
          frame No Error {
          }
          frame Error {
          }
        }
      }
      frame "Finish", Default {
        n179 = property on="Stop Chart" class="Bool (strict)"("Val(Sgnl)"=TRUE ("Value (Signaling)")) -> ()  [unwired: 2 in, 2 out]
        n180 = property on="Chart Data" class="Bool (strict)"("Val(Sgnl)"=FALSE ("Chart Data")) -> ()  [unwired: 2 in, 2 out]
        n181 = case shown="No Error" w448 {
          selector: w448 -> [w452 w454]
          tunnel: [w453 w455] -> w451
          tunnel: w450 -> [w453 w455]
          tunnel: [w452 w454] -> w449
          frame No Error {
          }
          frame Error {
          }
        }
      }
    }
    n182 = Equal?(x=w28, y="Finish") -> (x = y?=w36:bool)
  }
  n183 = while {
    tunnel: "Equipment" -> [w459]
    tunnel: w3 -> [w458]
    tunnel: w2 -> [w456]
    tunnel: w1 -> [_]
    stop <- "Stop Chart" stop-if-true
    n184 = Wait (ms)(milliseconds to wait=u32 1000) -> ()  [unwired: 1 out]
    n185 = case shown="True" "Chart Data" {
      tunnel: w459 -> [_ w466]
      tunnel: w458 -> [_ w465]
      tunnel: w456 -> [_ w462]
      frame False {
      }
      frame True {
        w468 = T8[] [37, 17] items=["4-20_OUT", "Pres_HI1", "Pres_HI2", "Pres_LOW", "Pres_PIN", "HEATER_TOP", "HEATER_BOT", "T_Shell", "FLOWMETER", "WATT_SENSE", "WH_TICK", "Tc_1", "Tc_2", "Tc_3", "Tc_4", "Tc_5", "Tc_6", "Tc_down", "T_Shell_2", "T_Shell_3", "T_Shell_4", "RTD_IN", "RTD_OUT", "RTD_AMB", "INTF_TEMPFLO", "INTF_READY", "INTF_START", "INTF_STOP", "DRM_LOW", "DRM_HIGH", "PWR_MAIN", "VLV_DUMP", "VLV_OUT", "VLV_IN", "WATT_HOURS", "FLOW(SAMPLE)", "GALLONS", "FLOW(GPM)"]
        n186 = Unbundle By Name(w466) -> ("MW100"=w467:refnum<visa-resource-name>)
        n187 = for {
          tunnel: w467 -> [w479]
          tunnel: w465 -> [w478]
          tunnel: w468 -> [w477] mode=indexing
          tunnel: [w476] -> w469 mode=indexing
          n188 = call "Generic - AI1.vi"("MW100"=w479, "Semiphore"=w478, "Channel_Enum"=w477) -> ("Value"=w476:dbl)  [unwired: 10 in, 2 out]
        }
        n189 = Index Array(array=w469, index #1=0 ("index"), index #2=1 ("index")) -> (element #1=w464:dbl, element #2=w463:dbl)
        n190 = local write "Downspout Flow Chart"(w464) -> ()
        n191 = local write "Downspout Temp Chart"(w463) -> ()
        n192 = case shown="False" w462 {
          tunnel: w464 -> [w475 _]
          tunnel: w463 -> [w473 _]
          frame False {
            n193 = property on="Property Node" class="WFChart (strict)"(reference="Flow Chart Ref", "Value"=w475) -> ()  [unwired: 1 in, 2 out]
            n194 = property on="Property Node" class="WFChart (strict)"(reference="Temp Chart Ref", "Value"=w473) -> ()  [unwired: 1 in, 2 out]
          }
          frame True {
          }
        }
      }
    }
  }
  n195 = call "Semiphore-Destroy-Local.vi"("Semiphore"=w7, "Local?"=w2, "error in (no error)"=w9) -> ("error out"=→"Error Out":errorcluster)  [unwired: 16 in]
